vi "Exercise 2.15.vi"() -> ()   [LabVIEW 2020]
panel:
  out "LED 6":bool=TRUE
  out "LED 5":bool=TRUE
  out "LED 4":bool=TRUE
  out "LED 3":bool=TRUE
  out "LED 2":bool=TRUE
  out "LED 1":bool=TRUE
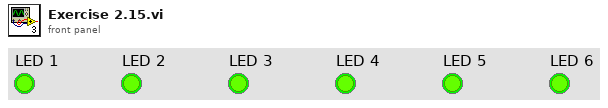
[diagram p1: front panel]
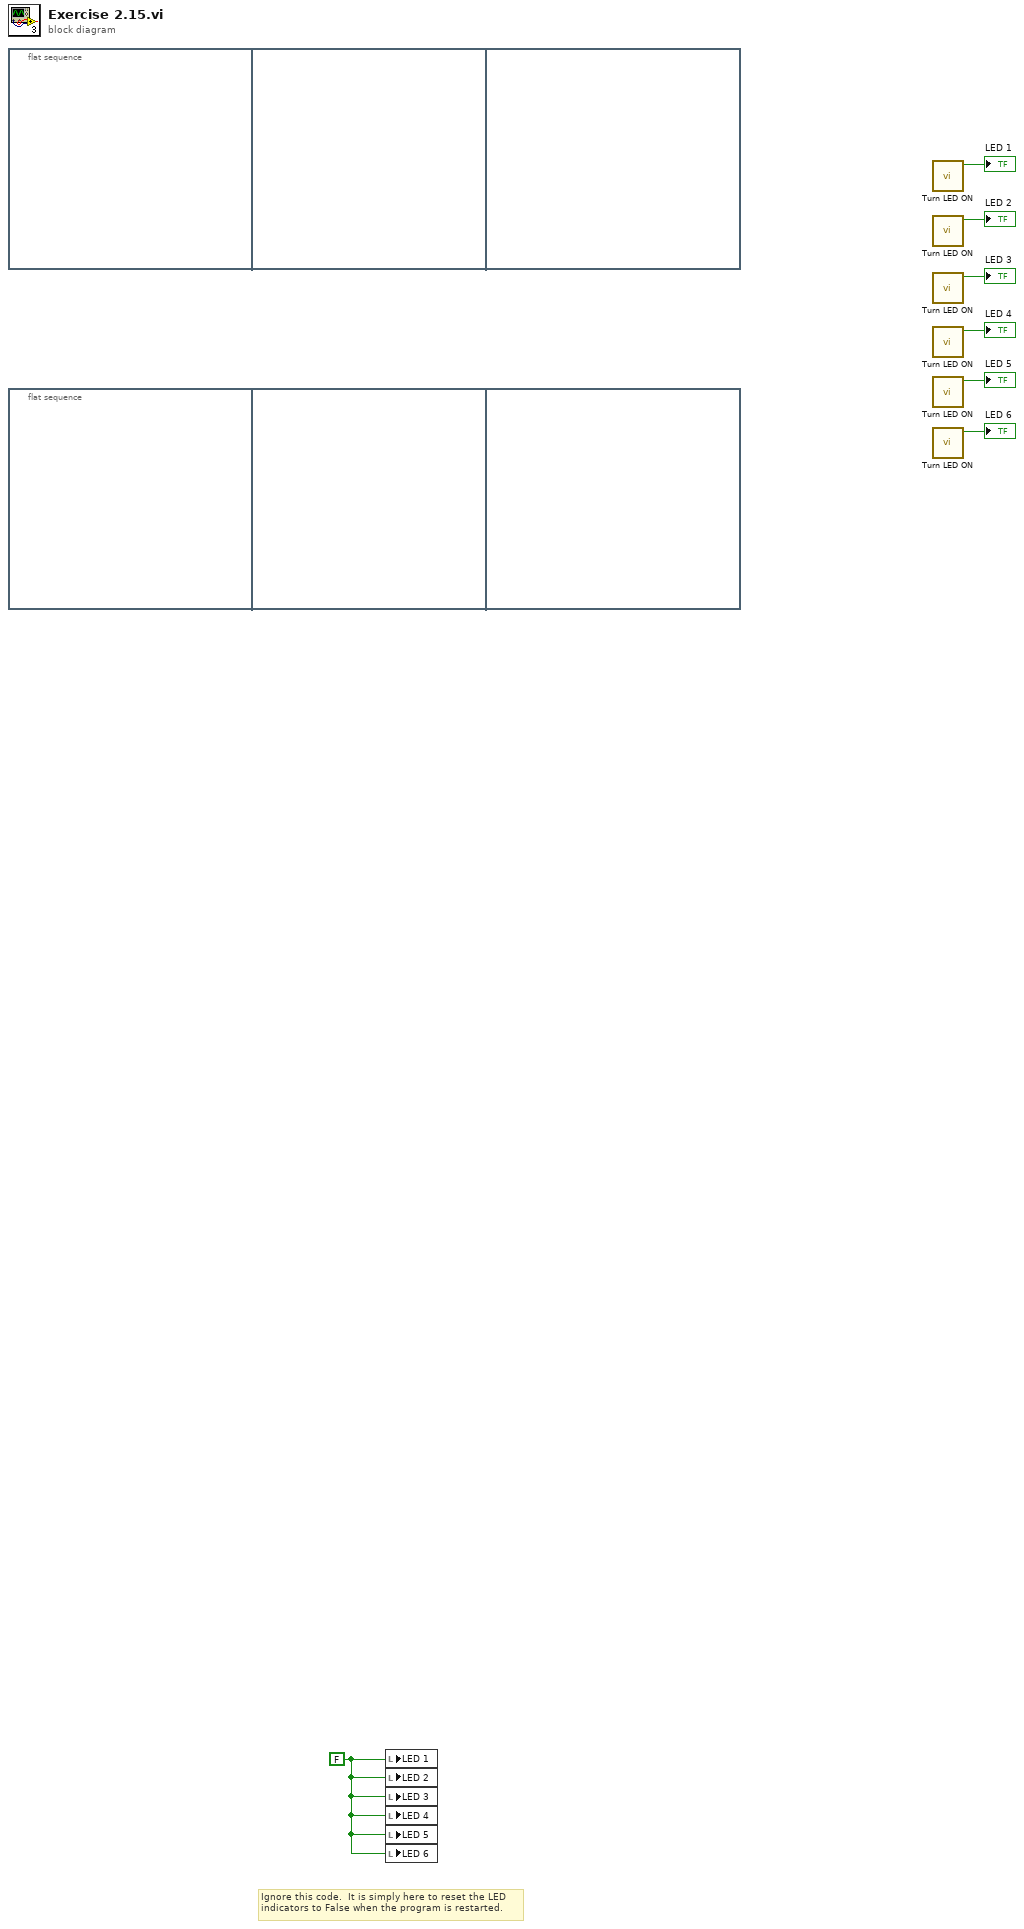
[diagram p0: block diagram]
diagram:
  w1 = FALSE
  # "Ignore this code.  It is simply here to reset the LED\nindicators to False when the program is restarted."
  n1 = flat-sequence {
    frame #0 {
    }
    frame #1 {
    }
    frame #2 {
    }
  }
  n2 = flat-sequence {
    frame #0 {
    }
    frame #1 {
    }
    frame #2 {
    }
  }
  n3 = local write "LED 1"(w1) -> ()
  n4 = local write "LED 2"(w1) -> ()
  n5 = local write "LED 3"(w1) -> ()
  n6 = local write "LED 4"(w1) -> ()
  n7 = local write "LED 5"(w1) -> ()
  n8 = local write "LED 6"(w1) -> ()
  n9 = call "Turn LED ON.vi"() -> ("Boolean"=→"LED 1":bool)  [unwired: 11 in]
  n10 = call "Turn LED ON.vi"() -> ("Boolean"=→"LED 2":bool)  [unwired: 11 in]
  n11 = call "Turn LED ON.vi"() -> ("Boolean"=→"LED 3":bool)  [unwired: 11 in]
  n12 = call "Turn LED ON.vi"() -> ("Boolean"=→"LED 4":bool)  [unwired: 11 in]
  n13 = call "Turn LED ON.vi"() -> ("Boolean"=→"LED 5":bool)  [unwired: 11 in]
  n14 = call "Turn LED ON.vi"() -> ("Boolean"=→"LED 6":bool)  [unwired: 11 in]
